vi "dataAcquiqition_back.vi"(0 "Background image handle":u32, 1 "Image Handle":u32, 2 "Camera Handle":u32, 3 "Error IN":errorcluster caption="entrée d'erreur (pas d'erreur)", 4 "Strip number":u32) -> (7 "Camera handle":i32, 8 "Image Handle":u32, 10 "Error OUT":errorcluster caption="sortie d'erreur")   [LabVIEW 2020]
panel:
  in  "SITKFULLDISPLAYLib.SITKFullDisplay":refnum<k7>(container)
  in  "Use background":bool
  out "Graphe":u16[][](graph)
  in  "Stop acquisiton":bool
  # "Strips spectral"
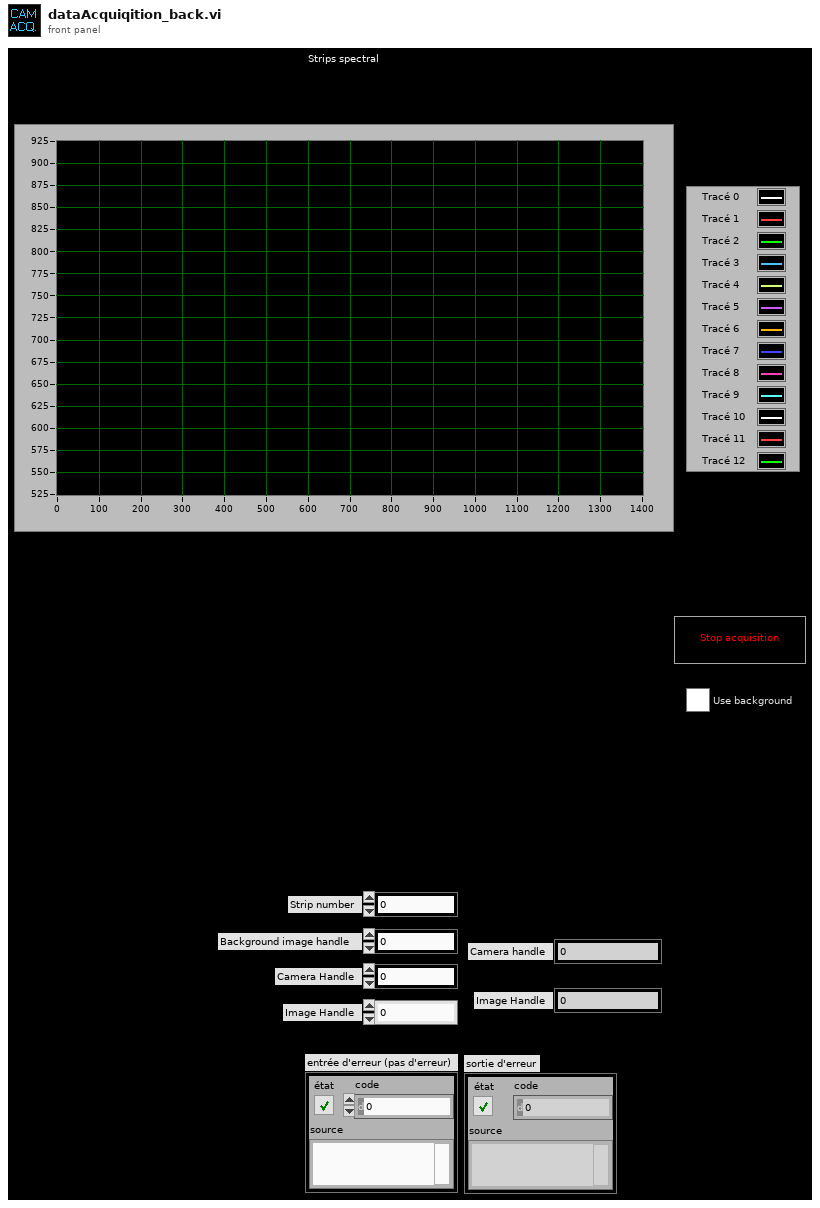
[diagram p1: front panel]
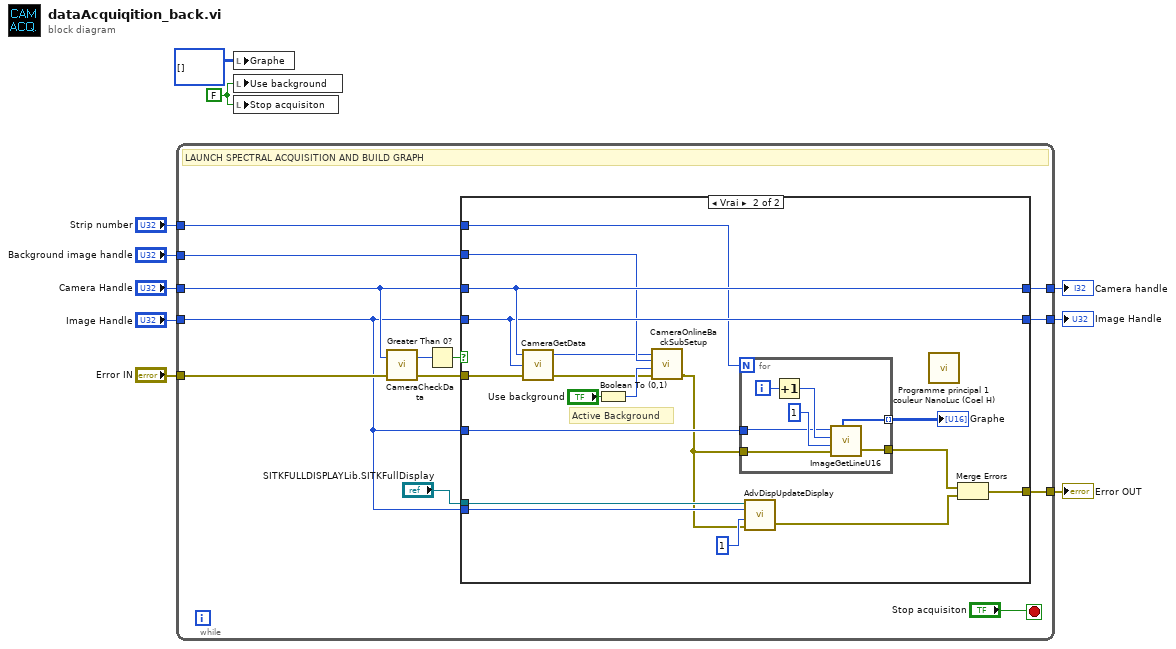
[diagram p0: block diagram]
diagram:
  w5 = FALSE ("Stop acquisiton")
  n1 = while {
    tunnel: "Error IN" -> [w15]
    tunnel: "Image Handle" -> [w11]
    tunnel: "Camera Handle" -> [w13]
    tunnel: [w21] -> w8
    tunnel: [w20] -> w10
    tunnel: [w19] -> w9
    tunnel: "Background image handle" -> [w14]
    tunnel: "Strip number" -> [w12]
    stop <- "Stop acquisiton" stop-if-true
    # "LAUNCH SPECTRAL ACQUISITION AND BUILD GRAPH"
    n2 = call <userlib>:"CameraCheckData.vi"("Camera Handle"=w13, "error in"=w15) -> ("Number Of Frames Available"=w16:i32, "error out"=w23:errorcluster)  [unwired: 1 out]
    n3 = Greater Than 0?(x=w16) -> (x > 0?=w22:bool)
    n4 = case shown="Vrai" w22 {
      tunnel: w23 -> [w26 w44]
      tunnel: w11 -> [w24 w37]
      tunnel: w13 -> [w25 w38]
      tunnel: [w26 w28] -> w21
      tunnel: [w25 w38] -> w20
      tunnel: [w24 w37] -> w19
      tunnel: "SITKFULLDISPLAYLib.SITKFullDisplay" -> [_ w43]
      tunnel: w14 -> [_ w36]
      tunnel: w12 -> [_ w27]
      tunnel: w11 -> [_ w34]
      tunnel: w11 -> [_ w32]
      frame False {
      }
      frame True {
        # "Active Background"
        n5 = call <userlib>:"CameraGetData.vi"("error in"=w44, "Image/Data Handle"=w37, "Camera Handle"=w38) -> ("error out"=w39:errorcluster, "Camera Handle"=w33:u32)  [unwired: 1 out]
        n6 = Boolean To (0,1)(Boolean="Use background") -> (0, 1=w41:i16)
        n7 = call <userlib>:"CameraOnlineBackSubSetup.vi"("error in"=w39, "Background Flag"=w41, "Background Image Handle"=w36, "Camera Handle"=w33) -> ("error out"=w31:errorcluster)  [unwired: 2 out]
        n8 = for {
          N: w27 -> [_]
          tunnel: w32 -> [w48]
          tunnel: [w47] -> w35 mode=indexing
          tunnel: w31 -> [w46]
          tunnel: [w45] -> w30
          i -> [w51]
          n9 = Increment(x=w51) -> (x+1=w50:i32)
          n10 = call <userlib>:"ImageGetLineU16.vi"("Data Handle"=w48, "Y Position"=w50, "Z Position"=u32 1, "error in"=w46) -> ("Array u16"=w47:u16[], "error out"=w45:errorcluster)  [unwired: 1 out]
        }
        "Graphe" <- w35
        n11 = call <userlib>:"AdvDispUpdateDisplay.vi"("error in (no error)"=w31, "Frame Number To Display"=u32 1, "Image Handle"=w34, "SITKFULLDISPLAYLib.SITKFullDisplay"=w43) -> ("error out"=w29:errorcluster)  [unwired: 1 out]
        n12 = call "Programme principal 1 couleur NanoLuc (Coel H).vi"() -> ()  [unwired: 14 in, 2 out]
        n13 = Merge Errors(w30, w29) -> (w28:errorcluster)
      }
    }
  }
  "Camera handle" <- w10
  "Image Handle" <- w9
  "Error OUT" <- w8
  n14 = local write "Graphe"(i32[][] [] ("Graphe")) -> ()
  n15 = local write "Use background"(w5) -> ()
  n16 = local write "Stop acquisiton"(w5) -> ()
